vi "Step Core.vi"(8 "error in (no error)":errorcluster, 11 "Power Sweep in":refnum<class "Power Sweep.lvclass">) -> (0 "error out":errorcluster, 3 "Power Sweep out":refnum<class "Power Sweep.lvclass">)   [LabVIEW 2018, in "Power Sweep.lvlib" / "Power Sweep.lvclass"]
uses:
  Power Sweep.lvclass
  Plugins/TestStand API Tools (TSAT).lvlibp/Step Actions/TSAT Step Actions.lvlib
  Plugins/Measurement Interface.lvlibp/Measurement Interface.lvclass
  C:/Sequence Automation/Plugins/Measurement Interface.lvlibp/Measurement Interface.lvclass
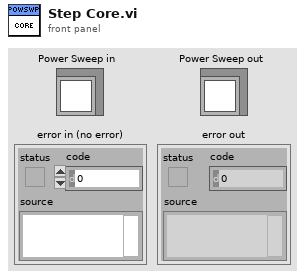
[diagram p1: front panel]
types:
  T1 = typedef "TestStand API Tools (TSAT).lvlibp/TSAT Evaluation Actions.lvlib/TSAT Evaluation.ctl" = cluster{"Test Name":string, "Pin":string, "Units":string, "SI Scaling":T2, "Test Number":i32, "Published Data Id":string, "Low Limit":dbl, "High Limit":dbl, "Export Data Location":string, "Software Bin":i64, "Evaluation Type":T3, "Test Data Source":string}
  T2 = typedef "TestStand API Tools (TSAT).lvlibp/TSAT Evaluation Actions.lvlib/TSAT Eval SI Unit Scaling.ctl" = i16
  T3 = typedef "TestStand API Tools (TSAT).lvlibp/TSAT Evaluation Actions.lvlib/TSAT Evaluation Type.ctl" = enum16{"Numeric Limit", "Pass/Fail", "None"}
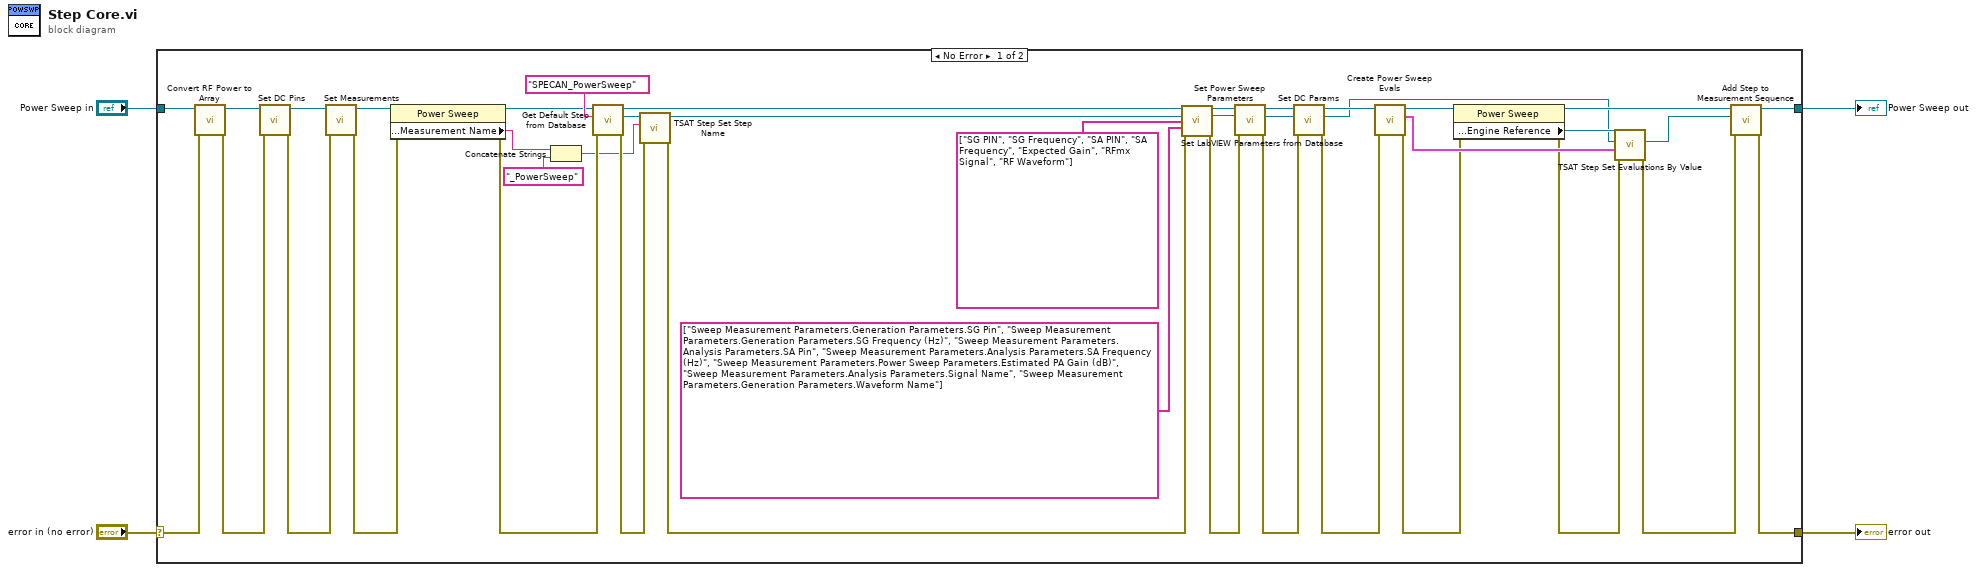
[diagram p0: block diagram]
diagram:
  n1 = case shown="No Error" "error in (no error)" {
    selector: "error in (no error)" -> [w37 w46]
    tunnel: [w16 w46] -> w3
    tunnel: [w28 w45] -> w1
    tunnel: "Power Sweep in" -> [w38 w45]
    frame No Error {
      n2 = call "Convert RF Power to Array.vi"("error in (no error)"=w37, "ModSweep in"=w38) -> ("error out"=w36:errorcluster, "ModSweep out"=w17:refnum<class "Power Sweep.lvclass">)  [unwired: 8 in]
      n3 = call "Set DC Pins.vi"("error in (no error)"=w36, "Power Sweep In"=w17) -> ("error out"=w6:errorcluster, "Power Sweep Out"=w8:refnum<class "Power Sweep.lvclass">)  [unwired: 8 in]
      n4 = call "Set Measurements.vi"("error in (no error)"=w6, "Power Sweep in"=w8) -> ("error out"=w5:errorcluster, "Power Sweep out"=w7:refnum<class "Power Sweep.lvclass">)  [unwired: 8 in]
      n5 = property class="Power Sweep"(reference=w7, error in=w5) -> (reference out=w21:refnum<class "Power Sweep.lvclass">, error out=w22:errorcluster, "Public Methods:Measurement Name"=w20:string)
      n6 = Concatenate Strings(w20, "_PowerSweep" ("string")) -> (w19:string)
      n7 = call "Get Default Step from Database.vi"("error in (no error)"=w22, "Default Step"="SPECAN_PowerSweep" ("FileGlobal to Clone"), "Measurement Interface in"=w21) -> ("error out"=w44:errorcluster, "Cloned Step"=w26:refnum<k7>, "Measurement Interface out"=w42:refnum<class "Power Sweep.lvclass">)  [unwired: 6 in]
      n8 = call "TSAT Step Set Step Name.vi"("Error In"=w44, "Name"=w19, "Step In"=w26) -> ("Error Out"=w27:errorcluster, "Step Out"=w25:refnum<k7>)  [unwired: 7 in]
      n9 = call "Set LabVIEW Parameters from Database.vi"("Measurement Interface in"=w42, "Step In"=w25, "Dictionary Keys"=string[] ["SG PIN", "SG Frequency", "SA PIN", "SA Frequency", "Expected Gain", "RFmx Signal", "RF Waveform"] ("Local Variable Mapping"), "LabVIEW Parameter Mapping"=string[] ["Sweep Measurement Parameters.Generation Parameters.SG Pin", "Sweep Measurement Parameters.Generation Parameters.SG Frequency (Hz)", "Sweep Measurement Parameters.Analysis Parameters.SA Pin", "Sweep Measurement Parameters.Analysis Parameters.SA Frequency (Hz)", "Sweep Measurement Parameters.Power Sweep Parameters.Estimated PA Gain (dB)", "Sweep Measurement Parameters.Analysis Parameters.Signal Name", "Sweep Measurement Parameters.Generation Parameters.Waveform Name"] ("Local Variable Mapping"), "error in (no error)"=w27) -> ("Measurement Interface out"=w35:refnum<class "Power Sweep.lvclass">, "Step Out"=w34:refnum<k7>, "error out"=w39:errorcluster)  [unwired: 8 in]
      n10 = call "Set Power Sweep Parameters.vi"("error in (no error)"=w39, "Step In"=w34, "ModSweep in"=w35) -> ("error out"=w10:errorcluster, "Step Out"=w12:refnum<k7>, "ModSweep out"=w14:refnum<class "Power Sweep.lvclass">)  [unwired: 6 in]
      n11 = call "Set DC Params.vi"("error in (no error)"=w10, "Step In"=w12, "Power Sweep in"=w14) -> ("error out"=w9:errorcluster, "Step Out"=w11:refnum<k7>, "Power Sweep out"=w13:refnum<class "Power Sweep.lvclass">)  [unwired: 6 in]
      n12 = call "Create Power Sweep Evals.vi"("error in (no error)"=w9, "ModSweep in"=w13) -> ("error out"=w32:errorcluster, "Evaluations Out"=w33:T1[], "ModSweep out"=w30:refnum<class "Power Sweep.lvclass">)  [unwired: 7 in]
      n13 = property class="Power Sweep"(reference=w30, error in=w32) -> (reference out=w24:refnum<class "Power Sweep.lvclass">, error out=w31:errorcluster, "Protected Methods:Engine Reference"=w29:refnum<k7>)
      n14 = call "TSAT Step Set Evaluations By Value.vi"("Error In"=w31, "Evaluation Data"=w33, "Step In"=w11, "Engine In"=w29) -> ("Error Out"=w15:errorcluster, "Step Out"=w23:refnum<k7>)  [unwired: 5 in, 1 out]
      n15 = call "Add Step to Measurement Sequence.vi"("error in (no error)"=w15, "Step to Add"=w23, "Measurement Interface in"=w24) -> ("error out"=w16:errorcluster, "Measurement Interface out"=w28:refnum<class "Power Sweep.lvclass">)  [unwired: 7 in]
    }
    frame Error {
    }
  }
  "error out" <- w3
  "Power Sweep out" <- w1
